vi "Check Installed.vi"(8 "error in (no error)":errorcluster, 11 "I Execution Adapter in":refnum<class "I Execution Adapter.lvclass">) -> (0 "error out":errorcluster, 3 "I Execution Adapter out":refnum<class "I Execution Adapter.lvclass">)   [LabVIEW 2026, in "I Execution Adapter.lvclass"]
uses:
  I Execution Adapter.lvclass
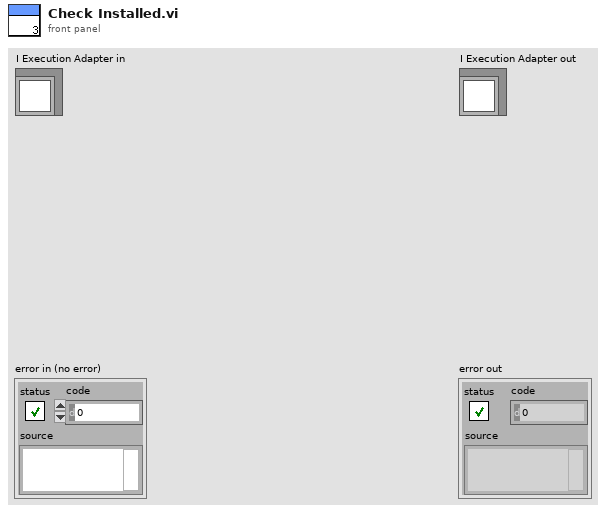
[diagram p1: front panel]
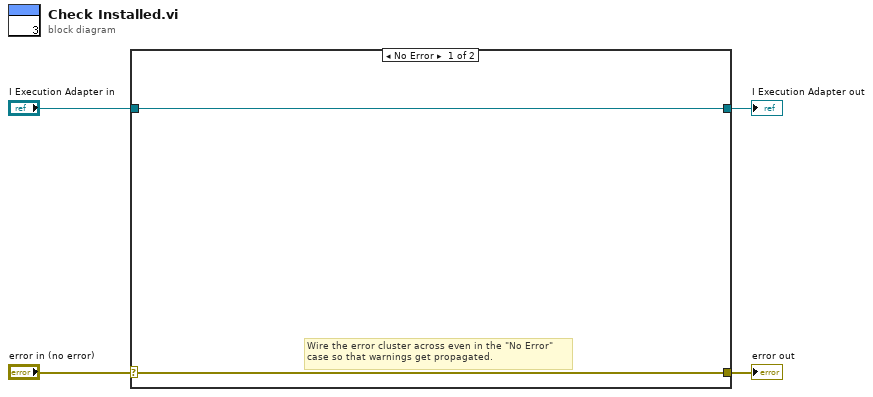
[diagram p0: block diagram]
diagram:
  n1 = case shown="No Error" "error in (no error)" {
    selector: "error in (no error)" -> [w5 w8]
    tunnel: [w5 w8] -> w3
    tunnel: [w6 w7] -> w1
    tunnel: "I Execution Adapter in" -> [w6 w7]
    frame No Error {
      # "Wire the error cluster across even in the \"No Error\"\ncase so that warnings get propagated."
    }
    frame Error {
    }
  }
  "error out" <- w3
  "I Execution Adapter out" <- w1
